vi "Get AccessType.vi"(8 "error in":errorcluster, 11 "DOMAIN in":refnum<class "DOMAIN.lvclass">) -> (0 "error out":errorcluster, 1 "Set?":bool, 2 "AccessType":enum16{"ro", "wo", "rw", "rwr", "rww", "const"}(ring)=enum."rw", 3 "DOMAIN out":refnum<class "DOMAIN.lvclass">)   [LabVIEW 2019, in "Electronic Datasheet.lvlib" / "DOMAIN.lvclass"]
uses:
  DOMAIN.lvclass
  Object Type/Object Type Base.lvclass
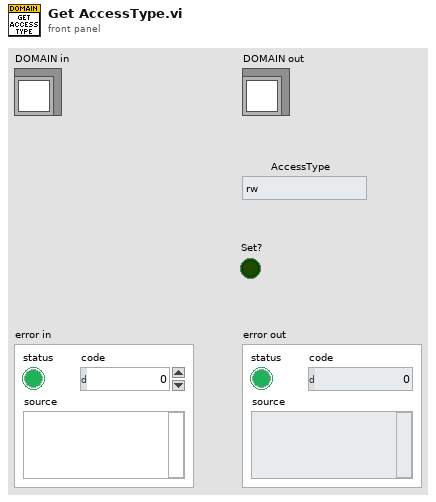
[diagram p1: front panel]
types:
  T1 = typedef "Electronic Datasheet.lvlib/Access Type.ctl" = enum16{"ro", "wo", "rw", "rwr", "rww", "const"}
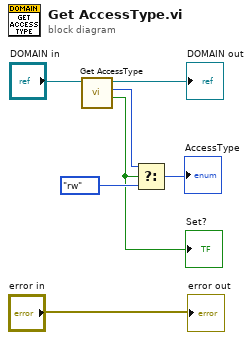
[diagram p0: block diagram]
diagram:
  n1 = call-parent "Get AccessType.vi"("Object Type in"="DOMAIN in") -> ("Defined?"=w2:bool, "AccessType"=w5:T1, "Object Type out"=→"DOMAIN out":refnum<class "DOMAIN.lvclass">)  [unwired: 7 in, 1 out]
  "Set?" <- w2
  n2 = Select(t=w5, s=w2, f=enum16{"ro", "wo", "rw", "rwr", "rww", "const"}."rw") -> (s? t:f=→"AccessType":T1)
  "error out" <- "error in"
